vi "execute.vi"(8 "error in (no error)":errorcluster, 9 "ParameterString":string, 10 "ObjectCluster":T1, 11 "TelevisionCommand in":refnum<class "TelevisionCommand.lvclass">) -> (0 "error out":errorcluster, 2 "ObjectCluster Out":T1, 3 "TelevisionCommand out":refnum<class "TelevisionCommand.lvclass">)   [LabVIEW 2013, in "TelevisionCommand.lvclass"]
uses:
  TelevisionCommand.lvclass
  Command.lvclass/ObjectCluster.ctl
  AirCondition.lvclass/AirCondition.lvclass
  RoomLight.lvclass/RoomLight.lvclass
  OutDoorLight.lvclass/OutDoorLight.lvclass
  Television.lvclass/Television.lvclass
  Stereo.lvclass/Stereo.lvclass
  Command.lvclass/Command.lvclass
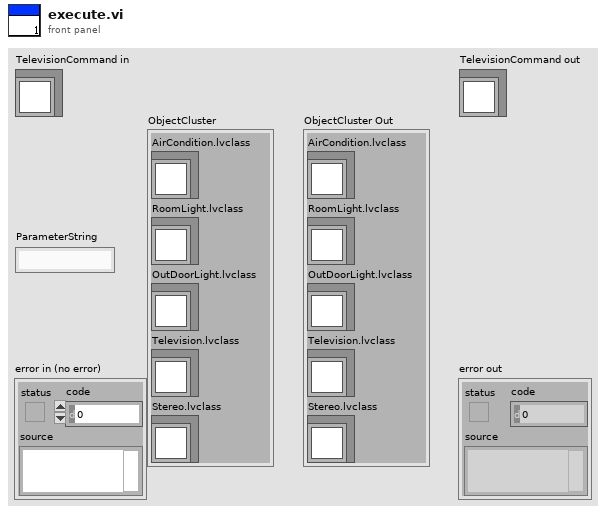
[diagram p1: front panel]
types:
  T1 = typedef "Command.lvclass/ObjectCluster.ctl" = cluster{"AirCondition.lvclass":refnum<class "AirCondition.lvclass">, "RoomLight.lvclass":refnum<class "RoomLight.lvclass">, "OutDoorLight.lvclass":refnum<class "OutDoorLight.lvclass">, "Television.lvclass":refnum<class "Television.lvclass">, "Stereo.lvclass":refnum<class "Stereo.lvclass">}
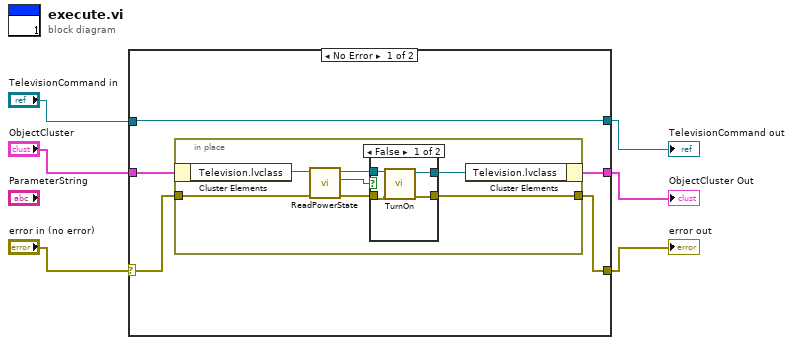
[diagram p0: block diagram]
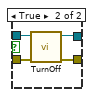
[diagram p2: hidden frame]
diagram:
  n1 = case shown="No Error" "error in (no error)" {
    selector: "error in (no error)" -> [w10 w27]
    tunnel: "ObjectCluster" -> [w11 w28]
    tunnel: "TelevisionCommand in" -> [w7 w29]
    tunnel: [w9 w27] -> w3
    tunnel: [w8 w28] -> w2
    tunnel: [w7 w29] -> w1
    frame No Error {
      n2 = in-place {
        in-place-border: w10 -> [w15]
        in-place-border: [w17] -> w9
        n3 = in-place-cluster #1(w11) -> ("Television.lvclass"=w16:refnum<class "Television.lvclass">)
        n4 = call-dynamic "ReadPowerState.vi"("error in (no error)"=w15, "Television in"=w16) -> ("error out"=w14:errorcluster, "PowerState"=w12:bool, "Television out"=w13:refnum<class "Television.lvclass">)  [unwired: 7 in]
        n5 = case shown="False" w12 {
          tunnel: w13 -> [w21 w25]
          tunnel: w14 -> [w22 w26]
          tunnel: [w20 w24] -> w18
          tunnel: [w19 w23] -> w17
          frame False {
            n6 = call-dynamic "TurnOn.vi"("error in (no error)"=w22, "Television in"=w21) -> ("error out"=w19:errorcluster, "Television out"=w20:refnum<class "Television.lvclass">)  [unwired: 8 in]
          }
          frame True {
            n7 = call-dynamic "TurnOff.vi"("error in (no error)"=w26, "Television in"=w25) -> ("error out"=w23:errorcluster, "Television out"=w24:refnum<class "Television.lvclass">)  [unwired: 8 in]
          }
        }
        n8 = in-place-cluster #1("Television.lvclass"=w18) -> (w8:T1)
      }
    }
    frame Error {
    }
  }
  "error out" <- w3
  "TelevisionCommand out" <- w1
  "ObjectCluster Out" <- w2
